vi "Meas - Filter Meas VI names.vi"(8 "error in":errorcluster, 10 "filenames In":string[](array[string])) -> (0 "Error Out":errorcluster, 3 "Meas VIs Out":string[](array[string]))   [LabVIEW 2011]
doc: "This VI will filter the Meas VI names (which user has configure)."
uses:
  Controls/INIT- READ - WRITE.ctl
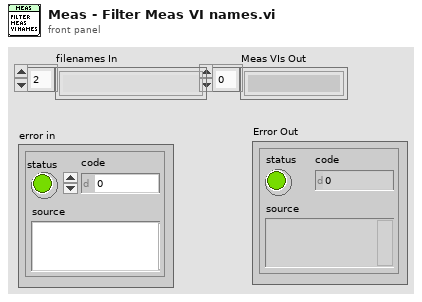
[diagram p1: front panel]
types:
  T1 = typedef "INIT- READ - WRITE.ctl" = enum16{"INIT", "READ", "WRITE"}
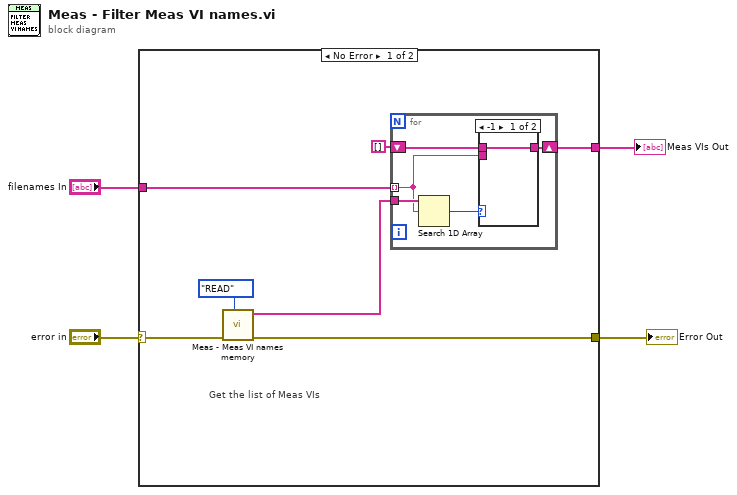
[diagram p0: block diagram]
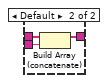
[diagram p2: hidden frame]
diagram:
  n1 = case shown="No Error" "error in" {
    selector: "error in" -> [w8 w21]
    tunnel: [w11 _] -> w4
    tunnel: "filenames In" -> [w9 _]
    tunnel: [w7 w21] -> w2
    frame No Error {
      # "Get the list of Meas VIs"
      n2 = call "Meas - Meas VI names memory.vi"("Operation"=INIT-_READ_-_WRITE."READ", "Error In"=w8) -> ("Error Out"=w7:errorcluster, "Names Out"=w6:string[])  [unwired: 8 in]
      n3 = for {
        tunnel: w9 -> [w15] mode=indexing
        tunnel: w6 -> [w16]
        shift-right: [w14] -> w11
        shift-left: string[] [] -> [w13]
        n4 = Search 1D Array(1D array=w16, element=w15) -> (index of element=w12:i32)  [unwired: 1 in]
        n5 = case shown="-1" w12 {
          tunnel: w15 -> [_ w20]
          tunnel: [w17 w19] -> w14
          tunnel: w13 -> [w17 w18]
          frame -1 {
          }
          frame Default {
            n6 = Build Array (concatenate)(w18, w20) -> (w19:string[])
          }
        }
      }
    }
    frame Error {
    }
  }
  "Meas VIs Out" <- w4
  "Error Out" <- w2
